vi "Agilent SNA Read Number of Available Traces.vi"(7 "Agilent SNA & SWP":T1, 8 "error in (no error)":errorcluster, 11 "VISA Resource Names":T2) -> (0 "error out":errorcluster, 2 "Number of Traces":i8, 3 "dup VISA Resource Names":T2)   [LabVIEW 2011]
doc: "This VI for the HP 8753 is used to read the sweep type.\n\n0 LINEAR FREQ\n1 LOG FREQ\n2 LIST FREQ\n3 CW TIME\n4 POWER SWEEP"
uses:
  TypeDefs/Agilent SNA VISA.ctl
  TypeDefs/Agilent SNA Instrument Info.ctl
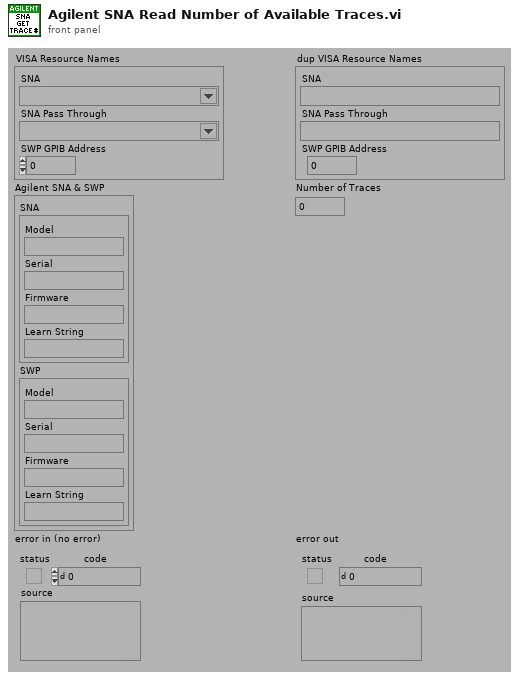
[diagram p1: front panel]
types:
  T1 = typedef "Agilent SNA Instrument Info.ctl" = cluster{"SNA":cluster{"Model":string, "Serial":string, "Firmware":string, "Learn String":string}, "SWP":cluster{"Model":string, "Serial":string, "Firmware":string, "Learn String":string}}
  T2 = typedef "Agilent SNA VISA.ctl" = cluster{"SNA":refnum<visa-resource-name>, "SNA Pass Through":refnum<visa-resource-name>, "SWP GPIB Address":i32}
  T3 = typedef "Agilent SNA Model.ctl" = enum16{"Not Supported", "8757X"}
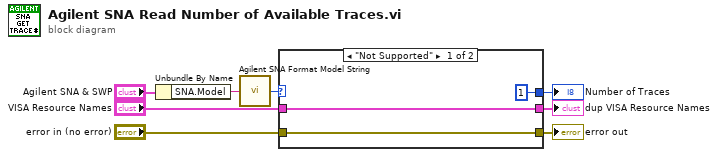
[diagram p0: block diagram]
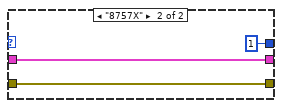
[diagram p2: hidden frame]
diagram:
  n1 = Unbundle By Name("Agilent SNA & SWP") -> ("SNA.Model"=w1:string)
  n2 = call "Agilent SNA Format Model String.vi"("Model String"=w1) -> ("Model"=w3:T3)
  n3 = case shown="\"Not Supported\"" w3 {
    tunnel: "VISA Resource Names" -> [w10 w12]
    tunnel: "error in (no error)" -> [w11 w13]
    tunnel: [w11 w13] -> w7
    tunnel: [i8 1 i8 1 ("Number of Channels")] -> w6
    tunnel: [w10 w12] -> w4
    frame "Not Supported" {
    }
    frame "8757X" {
    }
  }
  "Number of Traces" <- w6
  "dup VISA Resource Names" <- w4
  "error out" <- w7
